vi "Write Current.vi"(8 "error in":errorcluster, 10 "Current":dbl, 11 "89XX in":refnum<class "89XX.lvclass">) -> (0 "error out":errorcluster, 3 "89XX out":refnum<class "89XX.lvclass">)   [LabVIEW 2019, in "89XX.lvlib" / "89XX.lvclass"]
uses:
  Library/89XX.lvclass
  builds/Instruments/PowerSupply.lvlibp/Library/PowerSupply.lvclass
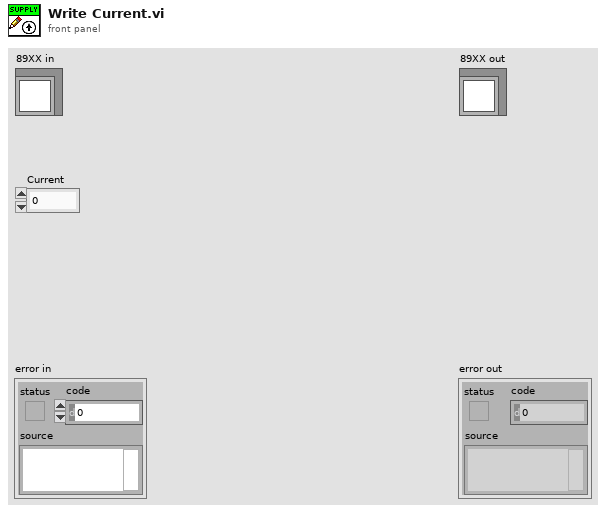
[diagram p1: front panel]
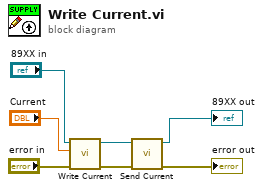
[diagram p0: block diagram]
diagram:
  n1 = call-parent "Write Current.vi"("error in"="error in", "Current"="Current", "PowerSupply in"="89XX in") -> ("error out"=w3:errorcluster, "PowerSupply out"=w4:refnum<class "89XX.lvclass">)  [unwired: 7 in]
  n2 = call "Send Current.vi"("error in"=w3, "89XX in"=w4) -> ("error out"=→"error out":errorcluster, "89XX out"=→"89XX out":refnum<class "89XX.lvclass">)  [unwired: 8 in]
